vi "Null Value.vi"() -> (0 "Null":variant)   [LabVIEW 2013, in "JKI JSON Serialization.lvlib"]
uses:
  JKI JSON Serialization.lvlib
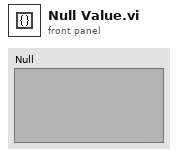
[diagram p1: front panel]
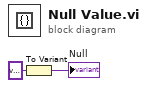
[diagram p0: block diagram]
diagram:
  n1 = To Variant(anything=variant ("variant")) -> (Variant=→"Null":variant)
